vi "test - Cluster with Reference.vi"(8 "error in (no error)":errorcluster, 11 "TestCase in":refnum<class "testcase-Supported-Datatype.lvclass">) -> (0 "error out":errorcluster, 3 "TestCase out":refnum<class "testcase-Supported-Datatype.lvclass">)   [LabVIEW 2017, in "testcase-Supported-Datatype.lvclass"]
uses:
  testcase-Supported-Datatype.lvclass
  7c75de9d-0fae-4e19-8970-b6a95c8ec96d.vi
  cc3e221a-1c58-402e-aa42-527ed3a1a0c0.vi
  43e9cd40-0bf7-4935-b2c6-3a97dc99e3f0.vi
  addons/API-String-Arugments-Support/_Support/Data To API String Arguments.vi
  <vilib>/addons/_JKI Toolkits/VI Tester/TestCase.llb/TestCase.lvclass
  C:/Program Files (x86)/National Instruments/LabVIEW 2017/vi.lib/addons/_JKI Toolkits/VI Tester/TestCase.llb/TestCase.lvclass
panel:
  out "String 3":string
  out "String 2":string
  out "String":string
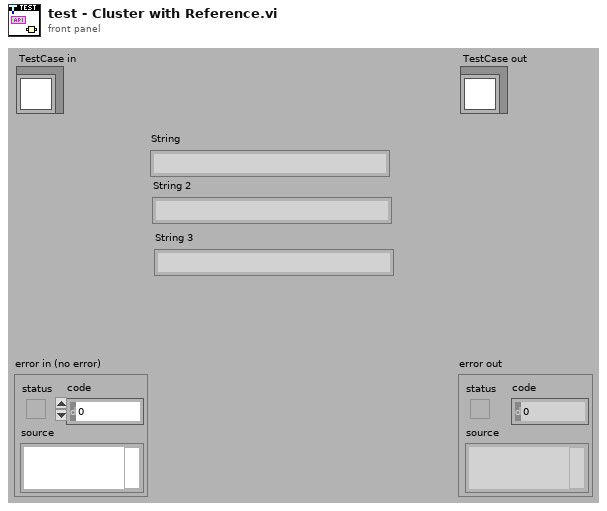
[diagram p1: front panel]
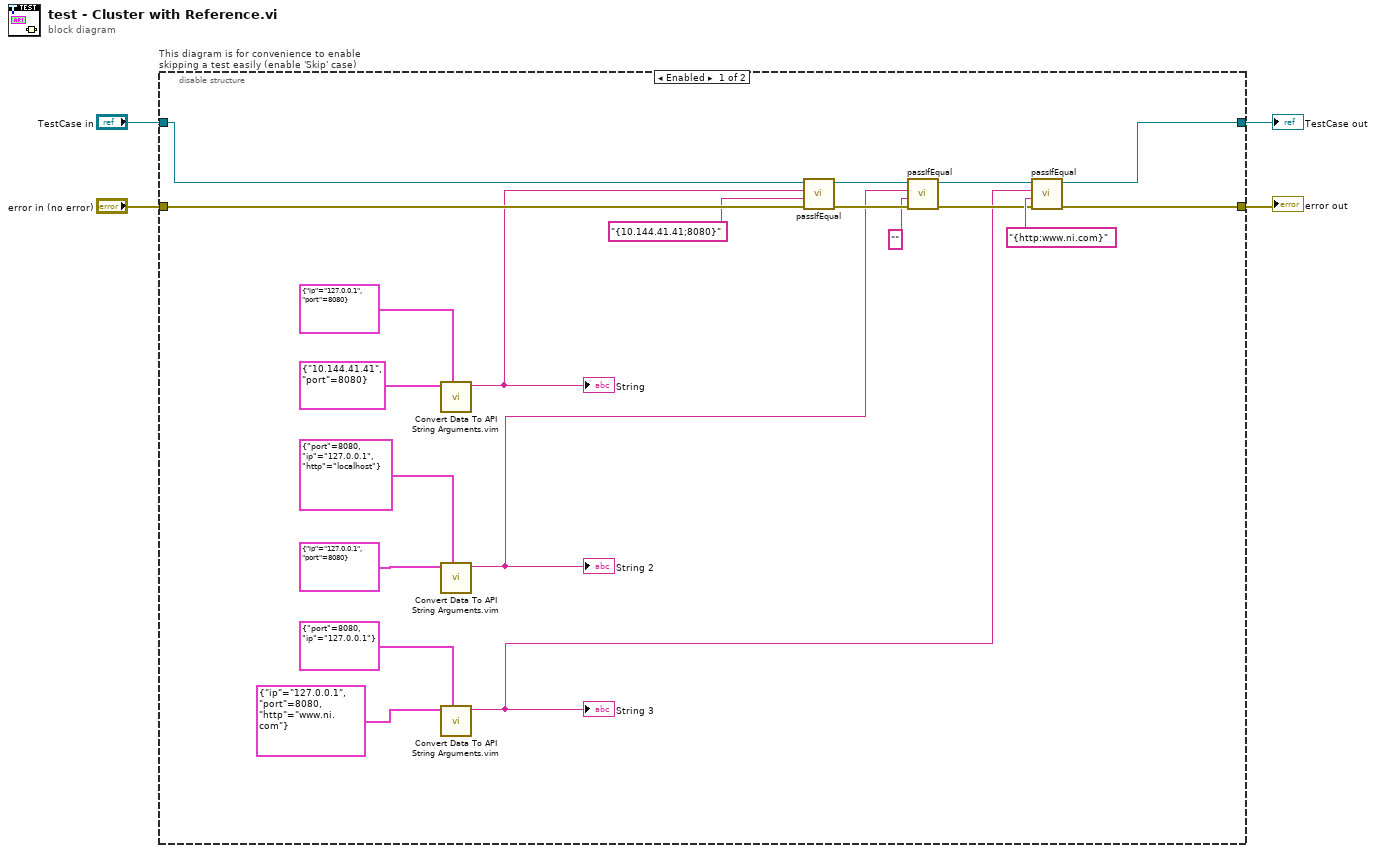
[diagram p0: block diagram]
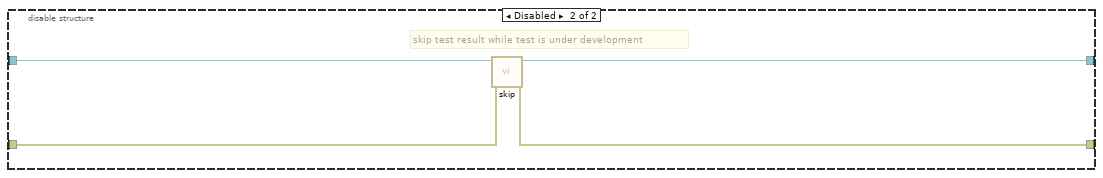
[diagram p2: hidden frame]
diagram:
  n1 = disable-structure "This diagram is for convenience to enable skipping a test easily (enable 'Skip' case)" shown="Enabled" {
    disable-tunnel: "TestCase in" -> [w24 w28]
    disable-tunnel: [w5 w26] -> w1
    disable-tunnel: [w9 w27] -> w3
    disable-tunnel: "error in (no error)" -> [w23 w25]
    frame Enabled {
      n2 = call "Convert Data To API String Arguments.vim"("Reference Cluster Data"=cluster{"ip":string, "port":i32} {"ip"="127.0.0.1", "port"=8080}, "Data"=cluster{string, "port":i32} {"10.144.41.41", "port"=8080}) -> ("API String"=w21:string)  [unwired: 6 in, 1 out]
      "String" <- w21
      n3 = call "Convert Data To API String Arguments.vim"("Reference Cluster Data"=cluster{"port":i32, "ip":string, "http":string} {"port"=8080, "ip"="127.0.0.1", "http"="localhost"}, "Data"=cluster{"ip":string, "port":i32} {"ip"="127.0.0.1", "port"=8080}) -> ("API String"=w14:string)  [unwired: 6 in, 1 out]
      "String 2" <- w14
      n4 = call "Convert Data To API String Arguments.vim"("Reference Cluster Data"=cluster{"port":i32, "ip":string} {"port"=8080, "ip"="127.0.0.1"}, "Data"=cluster{"ip":string, "port":i32, "http":string} {"ip"="127.0.0.1", "port"=8080, "http"="www.ni.com"}) -> ("API String"=w6:string)  [unwired: 6 in, 1 out]
      "String 3" <- w6
      n5 = call-dynamic "passIfEqual.vi"("error in (no error)"=w23, "y"="{10.144.41.41;8080}" ("String"), "x"=w21, "TestCase in"=w24) -> ("error out"=w15:errorcluster, "TestCase out"=w16:refnum<class "testcase-Supported-Datatype.lvclass">)  [unwired: 6 in]
      n6 = call-dynamic "passIfEqual.vi"("error in (no error)"=w15, "y"="" ("String"), "x"=w14, "TestCase in"=w16) -> ("error out"=w10:errorcluster, "TestCase out"=w11:refnum<class "testcase-Supported-Datatype.lvclass">)  [unwired: 6 in]
      n7 = call-dynamic "passIfEqual.vi"("error in (no error)"=w10, "y"="{http:www.ni.com}" ("String"), "x"=w6, "TestCase in"=w11) -> ("error out"=w9:errorcluster, "TestCase out"=w5:refnum<class "testcase-Supported-Datatype.lvclass">)  [unwired: 6 in]
    }
    frame Disabled {
      # "skip test result while test is under development"
      n8 = call <vilib>:"skip.vi"("error in (no error)"=w25, "TestCase in"=w28) -> ("error out"=w27:errorcluster, "TestCase out"=w26:refnum<class "testcase-Supported-Datatype.lvclass">)  [unwired: 8 in]
    }
  }
  "error out" <- w3
  "TestCase out" <- w1
